vi "Init.vi"(5 "Top Level VI":refnum<vi>, 7 "Config":T1={"Process Model"={"Seq Path"=""}, "Break On First Step?"=FALSE, "Break On Step Failure?"=TRUE, "Break On Sequence Failure?"=FALSE, "Tracing Enabled?"=TRUE, "Goto Cleanup on Sequence Failure?"=TRUE}, 8 "error in (no error)":errorcluster, 9 "Display Controls":T3, 10 "Manager Controls":T4, 11 "teststand-api in":refnum<class "teststand-api.lvclass">) -> (0 "error out":errorcluster, 3 "teststand-api out":refnum<class "teststand-api.lvclass">)   [LabVIEW 2014, in "teststand-api.lvlib" / "teststand-api.lvclass"]
uses:
  teststand-api.lvclass
  Manager Controls Argument--cluster.ctl
  TS Controls Argument--cluster.ctl
  Config Argument--cluster.ctl
  Process Model--cluster.ctl
  Other Refs Argument--cluster.ctl
  teststand-api.lvclass/teststand-api.ctl
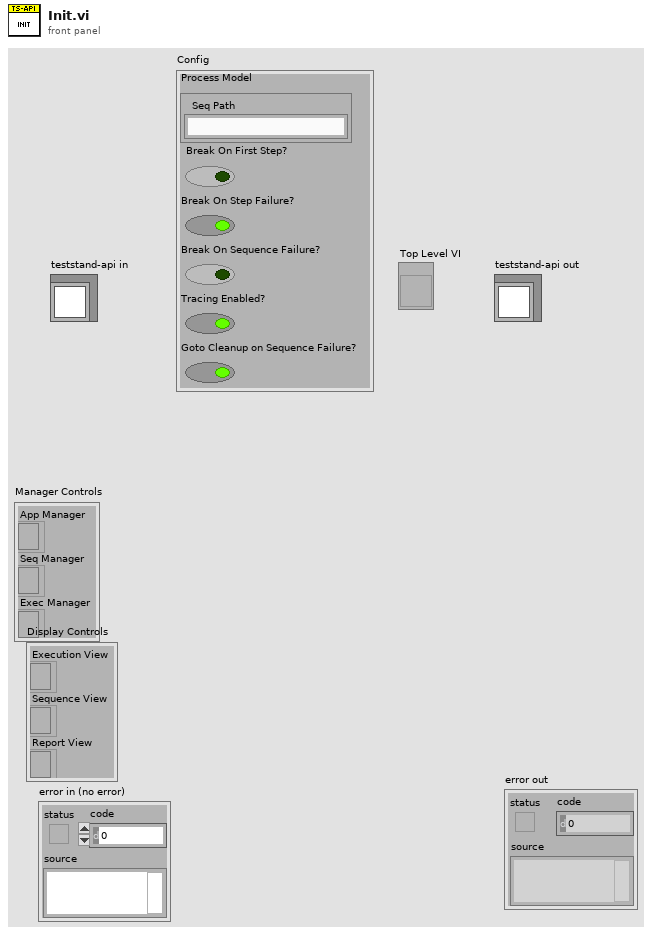
[diagram p1: front panel]
types:
  T1 = typedef "teststand-api.lvlib/teststand-api.lvclass/Config Argument--cluster.ctl" = cluster{"Process Model":T2, "Break On First Step?":bool, "Break On Step Failure?":bool, "Break On Sequence Failure?":bool, "Tracing Enabled?":bool, "Goto Cleanup on Sequence Failure?":bool}
  T2 = typedef "teststand-api.lvlib/teststand-api.lvclass/Process Model--cluster.ctl" = cluster{"Seq Path":string}
  T3 = typedef "teststand-api.lvlib/teststand-api.lvclass/TS Controls Argument--cluster.ctl" = cluster{"Execution View":refnum<k7>, "Sequence View":refnum<k7>, "Report View":refnum<k7>}
  T4 = typedef "teststand-api.lvlib/teststand-api.lvclass/Manager Controls Argument--cluster.ctl" = cluster{"App Manager":refnum<k7>, "Seq Manager":refnum<k7>, "Exec Manager":refnum<k7>}
  T5 = typedef "teststand-api.lvlib/teststand-api.lvclass/Other Refs Argument--cluster.ctl" = cluster{"TS Engine":refnum<k7>, "Top Level VI ":refnum<vi>, "Sequence File":refnum<k7>, "Execution":refnum<k7>, "Process Model Seq":refnum<k7>}
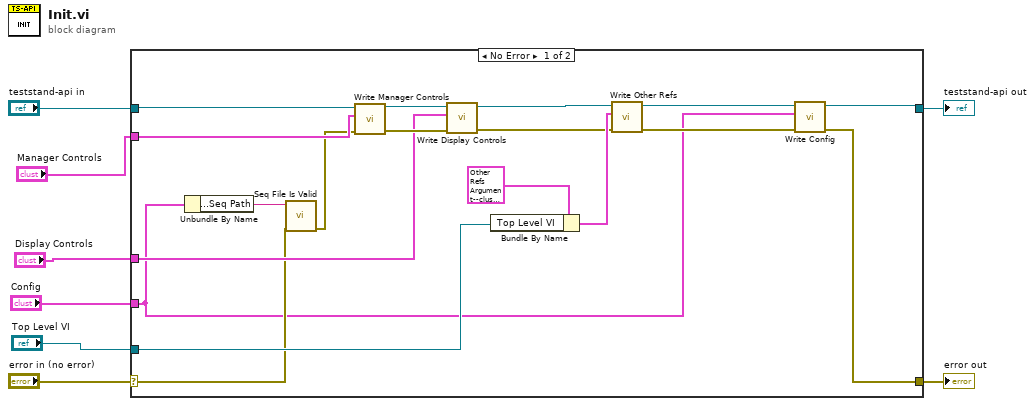
[diagram p0: block diagram]
diagram:
  n1 = case shown="No Error" "error in (no error)" {
    selector: "error in (no error)" -> [w10 w28]
    tunnel: [w15 w28] -> w7
    tunnel: [w14 w27] -> w5
    tunnel: "teststand-api in" -> [w26 w27]
    tunnel: "Manager Controls" -> [w25 _]
    tunnel: "Display Controls" -> [w22 _]
    tunnel: "Top Level VI" -> [w18 _]
    tunnel: "Config" -> [w9 _]
    frame No Error {
      n2 = Unbundle By Name(w9) -> ("Process Model.Seq Path"=w12:string)
      n3 = call "Seq File Is Valid.vi"("error in (no error)"=w10, "Seq File Path"=w12) -> ("error out"=w13:errorcluster)  [unwired: 9 in]
      n4 = call-dynamic "Write Manager Controls.vi"("error in (no error)"=w13, "Manager Controls"=w25, "teststand-api in"=w26) -> ("error out"=w23:errorcluster, "teststand-api out"=w24:refnum<class "teststand-api.lvclass">)  [unwired: 7 in]
      n5 = call-dynamic "Write Display Controls.vi"("error in (no error)"=w23, "Visible Controls"=w22, "teststand-api in"=w24) -> ("error out"=w17:errorcluster, "teststand-api out"=w21:refnum<class "teststand-api.lvclass">)  [unwired: 7 in]
      n6 = Bundle By Name(cluster=T5 {"TS Engine"=refnum, "Top Level VI "=refnum, "Sequence File"=refnum, "Execution"=refnum, "Process Model Seq"=refnum} ("Refs"), "Top Level VI"=w18) -> (w19:T5)
      n7 = call-dynamic "Write Other Refs.vi"("error in (no error)"=w17, "Refs"=w19, "teststand-api in"=w21) -> ("error out"=w11:errorcluster, "teststand-api out"=w16:refnum<class "teststand-api.lvclass">)  [unwired: 7 in]
      n8 = call "Write Config.vi"("error in (no error)"=w11, "Config"=w9, "teststand-api in"=w16) -> ("error out"=w15:errorcluster, "teststand-api out"=w14:refnum<class "teststand-api.lvclass">)  [unwired: 7 in]
    }
    frame Error {
    }
  }
  "error out" <- w7
  "teststand-api out" <- w5
